vi "Set Unzip File Date Time.vi"(7 "error in (no error)":errorcluster, 9 "Date_Time":T1, 10 "Path":path) -> (0 "error out":errorcluster)   [LabVIEW 2014, in "NI_Unzip.lvlib"]
uses:
  NI_Unzip.lvlib
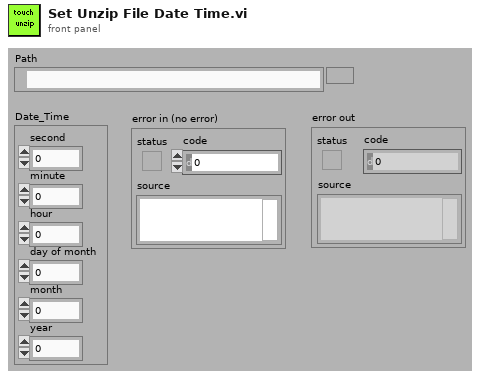
[diagram p1: front panel]
types:
  T1 = cluster{"second":u32, "minute":u32, "hour":u32, "day of month":u32, "month":u32, "year":u32}
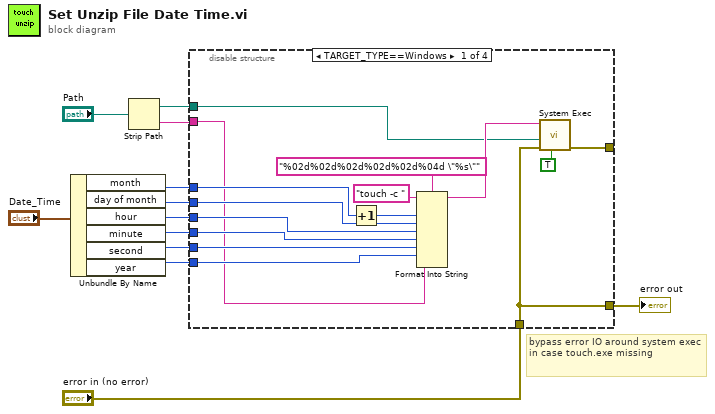
[diagram p0: block diagram]
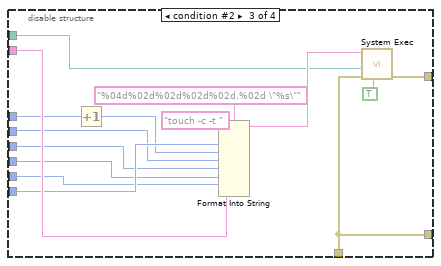
[diagram p3: hidden frame]
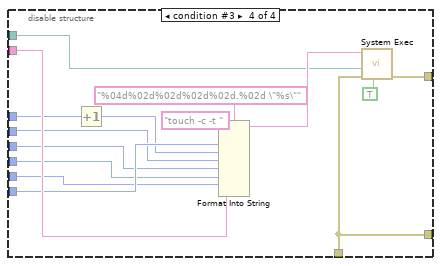
[diagram p4: hidden frame]
diagram:
  # "bypass error IO around system exec in case touch.exe missing"
  n1 = Unbundle By Name("Date_Time") -> ("month"=w11:u32, "day of month"=w10:u32, "hour"=w9:u32, "minute"=w8:u32, "second"=w7:u32, "year"=w6:u32)
  n2 = Strip Path(path="Path") -> (stripped path=w1:path, name=w4:string)
  n3 = disable-structure shown="TARGET_TYPE==Windows" {
    disable-tunnel: w11 -> [w27 _ w39 w54]
    disable-tunnel: w10 -> [w26 _ w37 w52]
    disable-tunnel: w9 -> [w25 _ w36 w51]
    disable-tunnel: w8 -> [w24 _ w35 w50]
    disable-tunnel: w7 -> [w23 _ w34 w49]
    disable-tunnel: w6 -> [w22 _ w40 w55]
    disable-tunnel: w4 -> [w19 _ w41 w56]
    disable-tunnel: "error in (no error)" -> [w14 w28 w29 w44]
    disable-tunnel: [w14 w28 w29 w44] -> w2
    disable-tunnel: w1 -> [w15 _ w31 w46]
    disable-tunnel: [w13 _ w30 w45] -> _
    frame condition #0 (active) {
      n4 = Increment(x=w27) -> (x+1=w18:u32)
      n5 = Format Into String(format string="%02d%02d%02d%02d%02d%04d \"%s\"", initial string="touch -c ", w18, w26, w25, w24, w23, w22, w19) -> (resulting string=w16:string)  [unwired: 1 in, 1 out]
      n6 = call "System Exec.vi"("run minimized? (F)"=TRUE, "error in (no error)"=w14, "working directory"=w15, "command line"=w16) -> ("error out"=w13:errorcluster)  [unwired: 4 in, 3 out]
    }
    frame condition #1 {
    }
    frame condition #2 {
      n7 = Increment(x=w39) -> (x+1=w38:u32)
      n8 = Format Into String(format string="%04d%02d%02d%02d%02d.%02d \"%s\"", initial string="touch -c -t ", w40, w38, w37, w36, w35, w34, w41) -> (resulting string=w32:string)  [unwired: 1 in, 1 out]
      n9 = call "System Exec.vi"("run minimized? (F)"=TRUE, "error in (no error)"=w29, "working directory"=w31, "command line"=w32) -> ("error out"=w30:errorcluster)  [unwired: 4 in, 3 out]
    }
    frame condition #3 {
      n10 = Increment(x=w54) -> (x+1=w53:u32)
      n11 = Format Into String(format string="%04d%02d%02d%02d%02d.%02d \"%s\"", initial string="touch -c -t ", w55, w53, w52, w51, w50, w49, w56) -> (resulting string=w47:string)  [unwired: 1 in, 1 out]
      n12 = call "System Exec.vi"("run minimized? (F)"=TRUE, "error in (no error)"=w44, "working directory"=w46, "command line"=w47) -> ("error out"=w45:errorcluster)  [unwired: 4 in, 3 out]
    }
  }
  "error out" <- w2
